vi "Set RPM.vi"(4 "Last Thrower Voltage (node)":dbl, 5 "Fine Tune?":bool, 6 "Position":dbl, 7 "Fine Tuning":dbl, 8 "EncoderDevRef":T8={"DevStatus"={"status"=FALSE, "code"=0, "source"=""}, "EncoderIndex"=enum."Invalid", "CounterIndex"=enum."Ctr 1", "DistancePerCount"=2.0, "Decoding Type"=enum."4x"}, 9 "Height":dbl, 11 "Distance":dbl) -> (0 "Thrower Voltage":dbl, 1 "RPM SET":bool, 3 "angle":dbl)   [LabVIEW 2011]
uses:
  <vilib>/Rock Robotics/WPI/Encoder/WPI_EncoderDevRef.ctl
  <vilib>/Rock Robotics/SystemInterfaces/Encoder/FPGA_EncoderIdx.ctl
  <vilib>/Rock Robotics/SystemInterfaces/Counter/FPGA_CounterCtrSystemIndex.ctl
  <vilib>/Rock Robotics/WPI/Encoder/WPI_EncoderType.ctl
  <vilib>/Rock Robotics/WPI/MotorControl/WPI_MotorControlDeviceRef.ctl
  <vilib>/Rock Robotics/SystemInterfaces/Typedef/FPGA_TypedefDigitalModule.ctl
  <vilib>/Rock Robotics/SystemInterfaces/DIO/FPGA_DIOPWMChannel.ctl
  <vilib>/Rock Robotics/WPI/PWM/WPI_PWMDeadband.ctl
  <vilib>/Rock Robotics/WPI/CAN/Jaguar/SubVIs/WPI_CANJaguar_ControlMode.ctl
  <vilib>/Rock Robotics/WPI/PWM/WPI_PWMTransform_ConPane.ctl
  <vilib>/Rock Robotics/WPI/CAN/Jaguar/SubVIs/WPI_CANJaguar_StatusSelect.ctl
panel:
  in  "CAN Slave":T1={"DeviceStatus"={"status"=FALSE, "code"=0, "source"=""}, "Type"=enum."PWM", "PWM"={"Digital Module"=enum."Digital Module 2", "PWM Channel"=enum."PWM 1", "DeadBand"={"Name"="", "maxPositivePwm"=0, "minPositivePwm"=0, "centerPwm"=0, "maxNegativePwm"=0, "minNegativePwm"=0, "angularRange"=0}}, "CAN"={"Device Number"=0, "Control Mode"=enum."Percent VBus", "Semaphore"=refnum, "Max Vout"=12.0}, "Invert"=FALSE, "TransformRef"=refnum, "InvTransformRef"=refnum}
  in  "CAN Master":T1={"DeviceStatus"={"status"=FALSE, "code"=0, "source"=""}, "Type"=enum."PWM", "PWM"={"Digital Module"=enum."Digital Module 2", "PWM Channel"=enum."PWM 1", "DeadBand"={"Name"="", "maxPositivePwm"=0, "minPositivePwm"=0, "centerPwm"=0, "maxNegativePwm"=0, "minNegativePwm"=0, "angularRange"=0}}, "CAN"={"Device Number"=0, "Control Mode"=enum."Percent VBus", "Semaphore"=refnum, "Max Vout"=12.0}, "Invert"=FALSE, "TransformRef"=refnum, "InvTransformRef"=refnum}
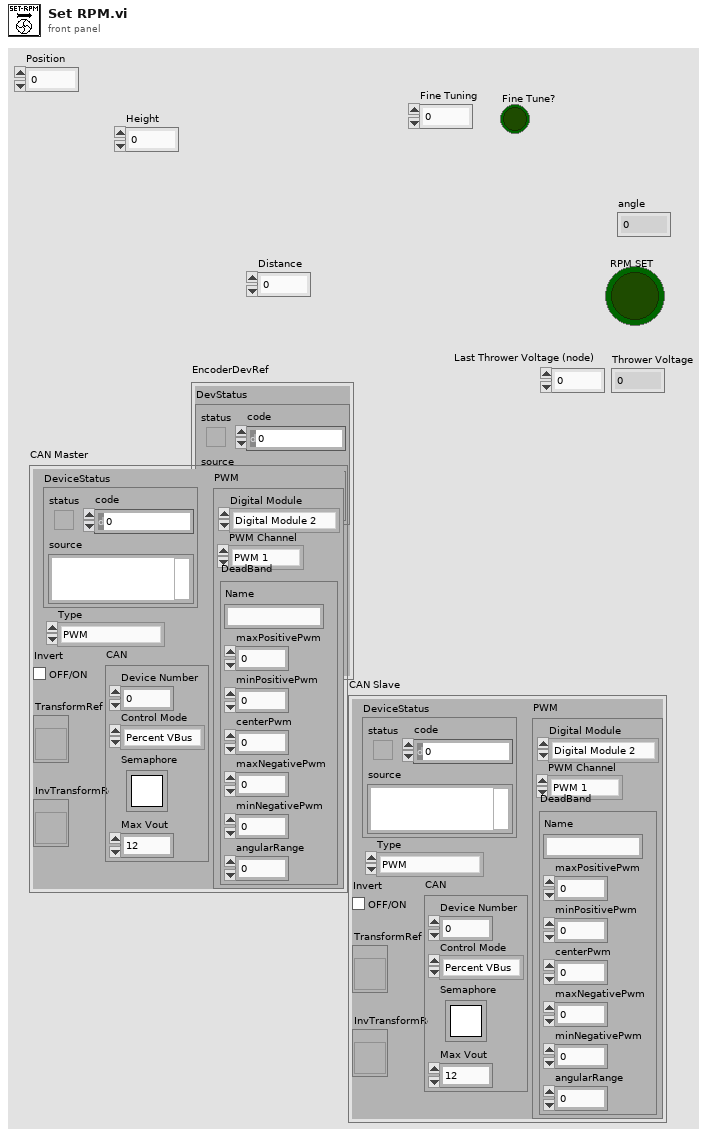
[diagram p1: front panel]
types:
  T1 = typedef "WPI_MotorControlDeviceRef.ctl" = cluster{"DeviceStatus":errorcluster, "Type":enum16{"PWM", "CAN"}, "PWM":cluster{"Digital Module":T2, "PWM Channel":T3, "DeadBand":T4}, "CAN":cluster{"Device Number":u8, "Control Mode":T5, "Semaphore":T6, "Max Vout":dbl}, "Invert":bool, "TransformRef":T7, "InvTransformRef":T7}
  T2 = typedef "FPGA_TypedefDigitalModule.ctl" = enum16{"Digital Module 1", "Digital Module 2"}
  T3 = typedef "FPGA_DIOPWMChannel.ctl" = enum8{"PWM 1", "PWM 2", "PWM 3", "PWM 4", "PWM 5", "PWM 6", "PWM 7", "PWM 8", "PWM 9", "PWM 10", "Invalid"}
  T4 = typedef "WPI_PWMDeadband.ctl" = cluster{"Name":string, "maxPositivePwm":i32, "minPositivePwm":i32, "centerPwm":i32, "maxNegativePwm":i32, "minNegativePwm":i32, "angularRange":u16}
  T5 = typedef "WPI_CANJaguar_ControlMode.ctl" = enum8{"Percent VBus", "Current", "Speed", "Position", "Voltage"}
  T6 = typedef "Semaphore RefNum" = refnum<k1>
  T7 = typedef "WPI_PWMTransform_ConPane.ctl" = refnum<vi>
  T8 = typedef "WPI_EncoderDevRef.ctl" = cluster{"DevStatus":errorcluster, "EncoderIndex":T9, "CounterIndex":T10, "DistancePerCount":dbl, "Decoding Type":T11}
  T9 = typedef "FPGA_EncoderIdx.ctl" = enum8{"Enc 0", "Enc 1", "Enc 2", "Enc 3", "Invalid"}
  T10 = typedef "FPGA_CounterCtrSystemIndex.ctl" = enum8{"Ctr 0", "Ctr 1", "Ctr 2", "Ctr 3", "Ctr 4", "Ctr 5", "Ctr 6", "Ctr 7", "Invalid"}
  T11 = typedef "WPI_EncoderType.ctl" = enum16{"1x", "2x", "4x"}
  T12 = typedef "WPI_CANJaguar_StatusSelect.ctl" = enum16{"Output Percent VBus", "Output Voltage", "Bus Voltage", "Current", "Temperature", "Position", "Speed", "Limit Switches", "Faults", "Fault Counters", "Power Cycle"}
  T13 = typedef "WPI_CANJaguar_Status.ctl" = cluster{"Output Percent VBus":dbl, "Output Voltage":dbl, "Bus Voltage":dbl, "Current":dbl, "Temperature":dbl, "Position":dbl, "Speed":dbl, "Limits":cluster{"Forward Limit":bool, "Reverse Limit":bool, "Forward Soft Limit":bool, "Reverse Soft Limit":bool, "Sticky Forward Limit":bool, "Sticky Reverse Limit":bool, "Sticky Forward Soft Limit":bool, "Sticky Reverse Soft Limit":bool}, "Faults":cluster{"Current Fault":bool, "Temperature Fault":bool, "Bus Voltage Fault":bool, "Gate Driver Fault":bool, "Comm Fault":bool}, "Fault Counters":cluster{"Current Faults":u8, "Temperature Faults":u8, "Bus Voltage Faults":u8, "Gate Driver Faults":u8, "Comm Faults":u8, "CAN Status":u8, "CAN RX Errors":u8, "CAN TX Errors":u8}, "Power Cycle":bool}
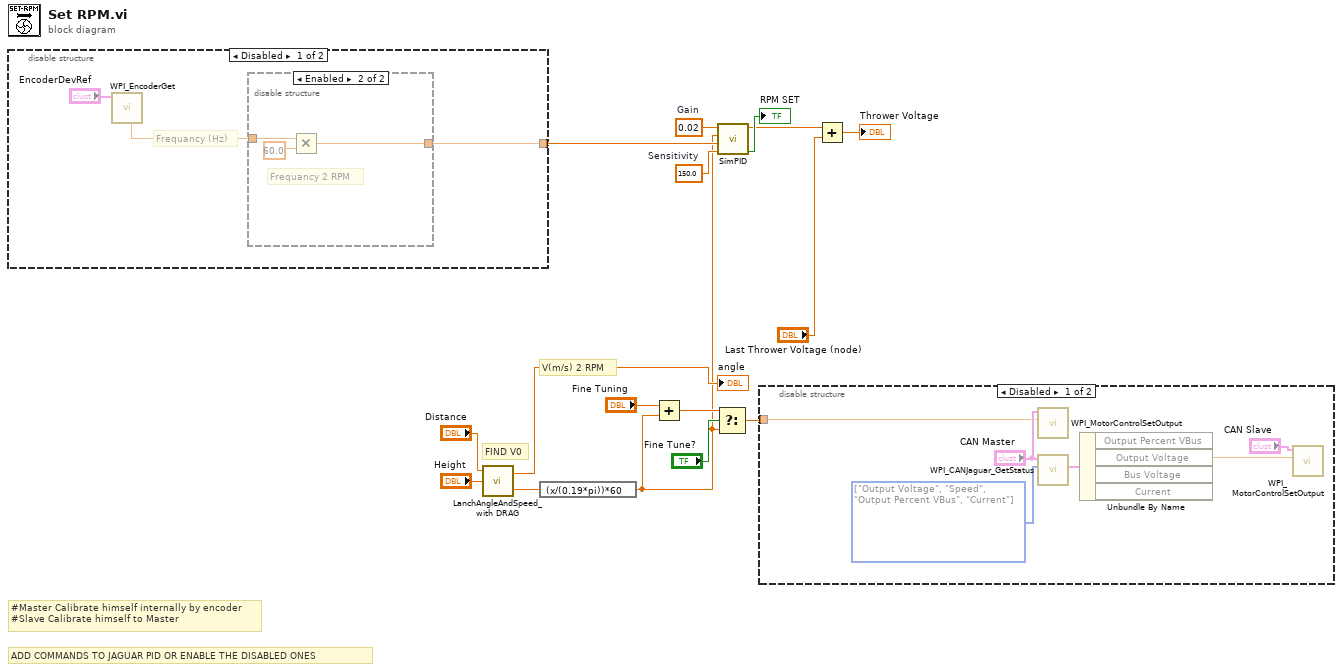
[diagram p0: block diagram]
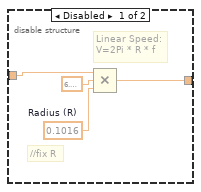
[diagram p3: hidden frame]
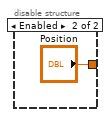
[diagram p4: hidden frame]
diagram:
  w4 = 0.02  # Gain
  w8 = 150.0  # Sensitivity
  # "#Master Calibrate himself internally by encoder\n#Slave Calibrate himself to Master"
  # "V(m/s) 2 RPM"
  # "ADD COMMANDS TO JAGUAR PID OR ENABLE THE DISABLED ONES"
  # "FIND V0"
  n1 = disable-structure shown="Disabled" {
    disable-tunnel: [w18 "Position"] -> w16
    frame Disabled {
      # "Frequancy (Hz)"
      n2 = call <vilib>:"WPI_EncoderGet.vi"("EncoderDevRef"="EncoderDevRef") -> ("Rate"=w19:dbl)  [unwired: 5 in, 5 out]
      n3 = disable-structure shown="Enabled" {
        disable-tunnel: w19 -> [w23 w26]
        disable-tunnel: [w20 w24] -> w18
        frame Disabled {
          w21 = 0.1016  # Radius (R)
          # "//fix R"
          # "Linear Speed:\nV=2Pi * R * f"
          n4 = Compound Arithmetic op=MULTIPLY(w23, 6.283185307179586, w21) -> (w20:dbl)
        }
        frame Enabled {
          # "Frequancy 2 RPM"
          n5 = Multiply(x=w26, y=60.0) -> (x*y=w24:dbl)
        }
      }
    }
    frame Enabled {
    }
  }
  n6 = call "LanchAngleAndSpeed_with DRAG.vi"("delta height (basket center-ball center) [m]"="Height", "distance to center of basket (x axies)"="Distance") -> ("initial velocity"=w13:dbl, "pitching angle"=→"angle":dbl)  [unwired: 1 in]
  n7 = expression code="(x/(0.19*pi))*60"(w13) -> (w5:dbl)
  n8 = Add(x="Fine Tuning", y=w5) -> (x+y=w10:dbl)
  n9 = Select(t=w10, s="Fine Tune?", f=w5) -> (s? t:f=w9:dbl)
  n10 = call "SimPID.vi"("Range"=w8, "Position"=w16, "Set Point"=w5, "Gain"=w4) -> ("On Target"=→"RPM SET":bool, "result"=w2:dbl)  [unwired: 5 in]
  n11 = disable-structure shown="Disabled" {
    disable-tunnel: w9 -> [w28 _]
    frame Disabled {
      w32 = T12[] [enum."Output Voltage", enum."Speed", enum."Output Percent VBus", enum."Current"] items=["Output Percent VBus", "Output Voltage", "Bus Voltage", "Current", "Temperature", "Position", "Speed", "Limit Switches", "Faults", "Fault Counters", "Power Cycle"] ("Status Select")
      n12 = call <vilib>:"WPI_MotorControlSetOutput.vi"("Output"=w28, "MotorControlDevRef"="CAN Master") -> ()  [unwired: 8 in, 2 out]
      n13 = call <vilib>:"WPI_CANJaguar_GetStatus.vi"("Status Select"=w32, "CAN Jaguar Ref"="CAN Master") -> ("Status"=w31:T13)  [unwired: 7 in, 2 out]
      n14 = Unbundle By Name(w31) -> ("Output Voltage"=w29:dbl)  [unwired: 3 out]
      n15 = call <vilib>:"WPI_MotorControlSetOutput.vi"("Output"=w29, "MotorControlDevRef"="CAN Slave") -> ()  [unwired: 8 in, 2 out]
    }
    frame Enabled {
    }
  }
  n16 = Add(x=w2, y="Last Thrower Voltage (node)") -> (x+y=→"Thrower Voltage":dbl)
